vi "TB-Save Setup Log.vi"(0 "State":T3, 1 "VI ref":refnum<vi>, 5 "Exposure parameters":T1={"Low cutoff (kHz)"=0.0, "High cutoff (kHz)"=0.0, "Duration (min)"=0.0, "dB SPL"=0.0, "Waveform"=enum."Noise", "WAVfile"=path "", "refWav"=path "", "use mic correction"=FALSE, "micCorrFile"=path "", "Pistonphone Level (dB SPL)"=0.0, "Sampling rate (Hz)"=0.0, "Buffer length (s)"=0.0, "Stream mic"=FALSE, "Fine adjust"={"Max"=0.0, "Min"=0.0}, "Mic gain"=0.0, "atten"=0.0, "Allow Slack"=FALSE, "max starts"=0, "Freq (kHz)"=8.0, "Tma (s)"=0.0, "Streamed"=[], "Drive"="", "Speaker"="", "Mic"="", "Analysis"={"Method"=enum."Default", "resol (Hz)"=0.0, "nfreq"=0, "signal"=""}}, 12 "Fine Control":dbl) -> (8 "date/time string":string, 15 "error out":errorcluster)   [LabVIEW 2020]
uses:
  Typedefs/TB-Runtime state.ctl
  <vilib>/sound2/lvsound2.llb/Sound File Refnum.ctl
  Typedefs/TB-Setup Log.ctl
  Typedefs/TB-Analysis State.ctl
  Typedefs/TB-Parameters.ctl
  Typedefs/TB-Analysis Parameters.ctl
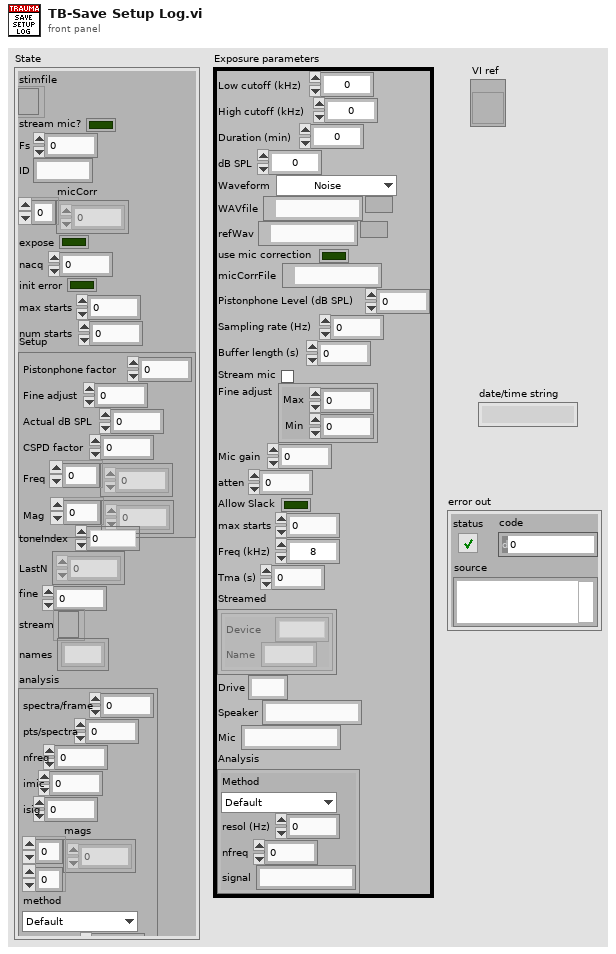
[diagram p1: front panel]
types:
  T1 = typedef "TB-Parameters.ctl" = cluster{"Low cutoff (kHz)":dbl, "High cutoff (kHz)":dbl, "Duration (min)":dbl, "dB SPL":dbl, "Waveform":enum16{"Noise", "File", "Tone"}, "WAVfile":path, "refWav":path, "use mic correction":bool, "micCorrFile":path, "Pistonphone Level (dB SPL)":dbl, "Sampling rate (Hz)":dbl, "Buffer length (s)":dbl, "Stream mic":bool, "Fine adjust":cluster{"Max":dbl, "Min":dbl}, "Mic gain":dbl, "atten":dbl, "Allow Slack":bool, "max starts":i32, "Freq (kHz)":dbl, "Tma (s)":dbl, "Streamed":cluster{"Device":string, "Name":string}[], "Drive":string, "Speaker":string, "Mic":string, "Analysis":T2}
  T2 = typedef "TB-Analysis Parameters.ctl" = cluster{"Method":enum16{"Default", "Periodogram", "Cross-spectrum"}, "resol (Hz)":dbl, "nfreq":i32, "signal":string}
  T3 = typedef "TB-Runtime state.ctl" = cluster{"stimfile":T4, "stream mic?":bool, "Fs":dbl, "ID":string, "micCorr":dbl[], "expose":bool, "nacq":i32, "init error":bool, "max starts":i32, "num starts":i32, "Setup":T5, "toneIndex":i32, "LastN":dbl[], "fine":dbl, "stream":refnum<file>, "names":string[], "analysis":T6}
  T4 = typedef "Sound File Refnum.ctl" = refnum<file>
  T5 = typedef "TB-Setup Log.ctl" = cluster{"Pistonphone factor":dbl, "Fine adjust":dbl, "Actual dB SPL":dbl, "CSPD factor":dbl, "Freq":dbl[], "Mag":dbl[]}
  T6 = typedef "TB-Analysis State.ctl" = cluster{"spectra/frame":i32, "pts/spectra":i32, "nfreq":i32, "imic":i32, "isig":i32, "mags":dbl[][], "method":enum16{"Default", "Periodogram", "Cross-spectrum"}, "cspd scale":dbl}
  T7 = typedef "imagedata.ctl" = cluster{"image type":i32, "image depth":i32, "image":u8[], "mask":u8[], "colors":u32[], "Rectangle":cluster{"left":i16, "top":i16, "right":i16, "bottom":i16}}
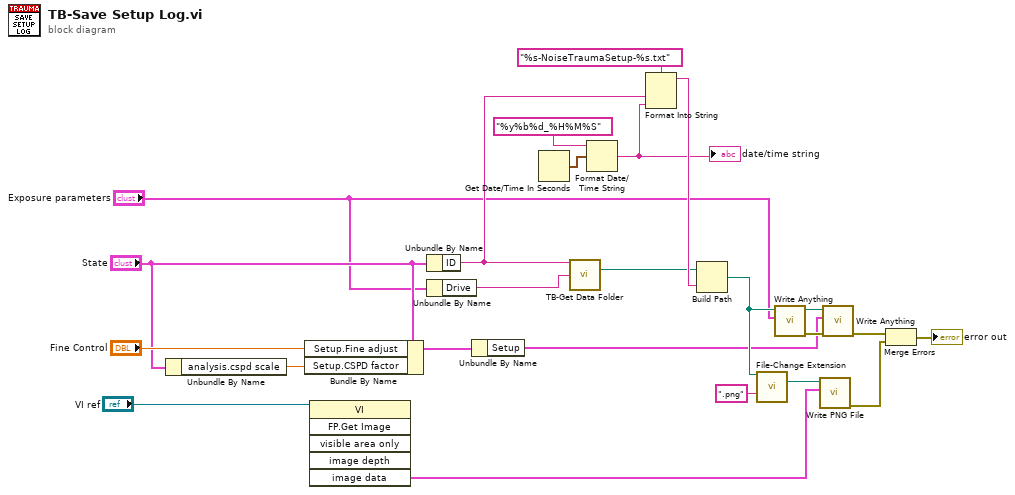
[diagram p0: block diagram]
diagram:
  n1 = Unbundle By Name("State") -> ("analysis.cspd scale"=w3:dbl)
  n2 = Bundle By Name(cluster="State", "Setup.Fine adjust"="Fine Control", "Setup.CSPD factor"=w3) -> (w18:T3)
  n3 = invoke class="VI" method="FP.Get Image"(reference="VI ref") -> ("image data"=w7:T7)  [unwired: 5 in, 5 out]
  n4 = Unbundle By Name("State") -> ("ID"=w5:string)
  n5 = Unbundle By Name("Exposure parameters") -> ("Drive"=w6:string)
  n6 = Unbundle By Name(w18) -> ("Setup"=w1:T5)
  n7 = Get Date/Time In Seconds() -> (seconds since 1Jan1904=w22:timestamp)
  n8 = call "TB-Get Data Folder.vi"("ID"=w5, "Drive"=w6) -> ("Data folder"=w13:path)  [unwired: 12 in, 1 out]
  n9 = Format Date/Time String(time format string (%c)="%y%b%d_%H%M%S", seconds (now)=w22) -> (date/time string=w20:string)  [unwired: 1 in]
  "date/time string" <- w20
  n10 = Format Into String(format string="%s-NoiseTraumaSetup-%s.txt", w5, w20) -> (resulting string=w23:string)  [unwired: 2 in, 1 out]
  n11 = Build Path(base path=w13, name or relative path=w23) -> (appended path=w12:path)
  n12 = call "File-Change Extension.vi"("Path"=w12, "new extension"=".png") -> ("new path"=w10:path)  [unwired: 12 in, 1 out]
  n13 = call "Write Anything.vi"("Anything"="Exposure parameters", "Path (dialog)"=w12) -> ("Error Out"=w16:errorcluster, "Path out"=w17:path)  [unwired: 8 in]
  n14 = call <vilib>:"Write PNG File.vi"("image data"=w7, "path to PNG file"=w10) -> ("error out"=w8:errorcluster)  [unwired: 8 in, 1 out]
  n15 = call "Write Anything.vi"("Error In"=w16, "Anything"=w1, "Path (dialog)"=w17) -> ("Error Out"=w15:errorcluster)  [unwired: 7 in, 1 out]
  n16 = Merge Errors(w15, w8) -> (→"error out":errorcluster)
